vi "getMessage.vi"(8 "error in (no error)":errorcluster, 11 "MonoClientCommunicator in":refnum<class "MonoClientCommunicator.lvclass">) -> (0 "error out":errorcluster, 2 "message":string, 3 "MonoClientCommunicator out":refnum<class "MonoClientCommunicator.lvclass">)   [LabVIEW 2016, in "MonoClientCommunicator.lvclass"]
uses:
  MonoClientCommunicator.lvclass
  MonoClientCommunicator.lvclass/MonoClientCommunicator.ctl
  ts_labview_tcp/TCPClient/TCPClient.lvclass
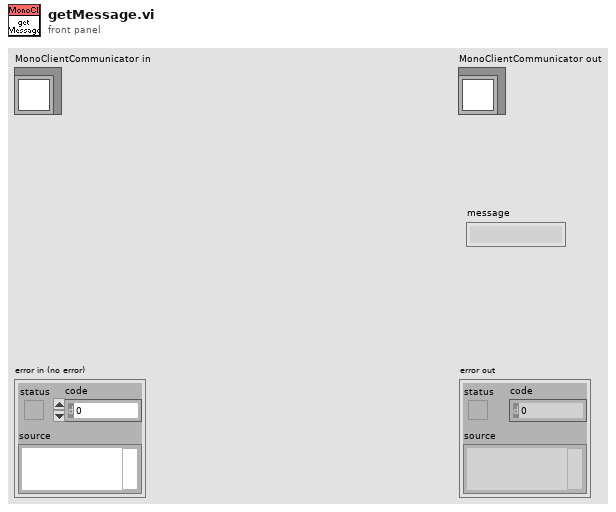
[diagram p1: front panel]
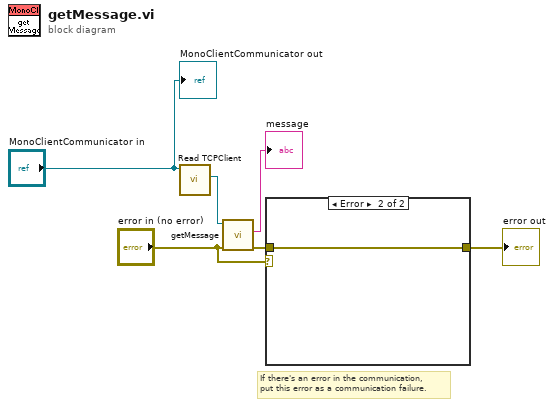
[diagram p0: block diagram]
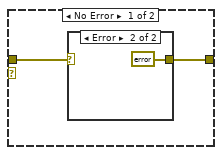
[diagram p2: hidden frame]
diagram:
  # "If there's an error in the communication, \nput this error as a communication failure."
  n1 = call "Read TCPClient.vi"("MonoClient in"="MonoClientCommunicator in") -> ("TCPClient.lvclass"=w5:refnum<class "TCPClient.lvclass">)  [unwired: 8 in, 2 out]
  n2 = call-dynamic "getMessage.vi"("error in (no error)"="error in (no error)", "TCPClient in"=w5) -> ("error out"=w2:errorcluster, "String"=→"message":string)  [unwired: 7 in, 1 out]
  n3 = case shown="Error" "error in (no error)" {
    tunnel: w2 -> [w8 w11]
    tunnel: [w7 w11] -> w1
    frame No Error {
      n4 = case shown="Error" w8 {
        selector: w8 -> [w9 _]
        tunnel: [w9 errorcluster {"status"=TRUE, "code"=8204, "source"="Monochromator Controller not responding"} ("error IO")] -> w7
        frame No Error {
        }
        frame Error {
        }
      }
    }
    frame Error {
    }
  }
  "error out" <- w1
  "MonoClientCommunicator out" <- "MonoClientCommunicator in"
